vi "rtout_getTriggerConfig.vi"(0 "connection ID":refnum<k5>, 1 "axis":i32, 2 "tempvalue":bool, 5 "error in":errorcluster) -> (12 "polarity":i32, 14 "connection ID":refnum<k5>, 15 "axis_out":i32, 16 "higher":i32, 17 "lower":i32, 18 "epsilon":i32, 19 "error out":errorcluster)   [LabVIEW 2016]
doc: "Get the real time output trigger config"
panel:
  out "params_cluster":cluster{"axis":i32, "tempvalue":bool}
  in  "Params_cluster":cluster{"integer":i32, "boolean":bool}
  in  "results_cluster":T1
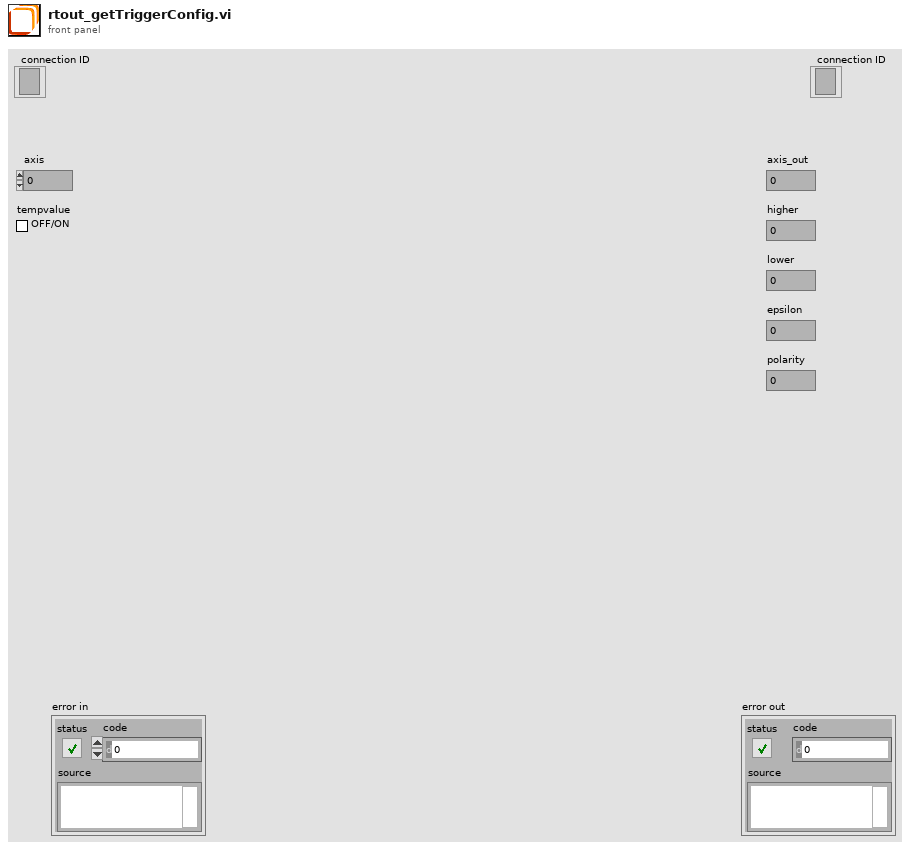
[diagram p1: front panel]
types:
  T1 = cluster{"errNo":i32, "higher":i32, "lower":i32, "epsilon":i32, "polarity":i32}
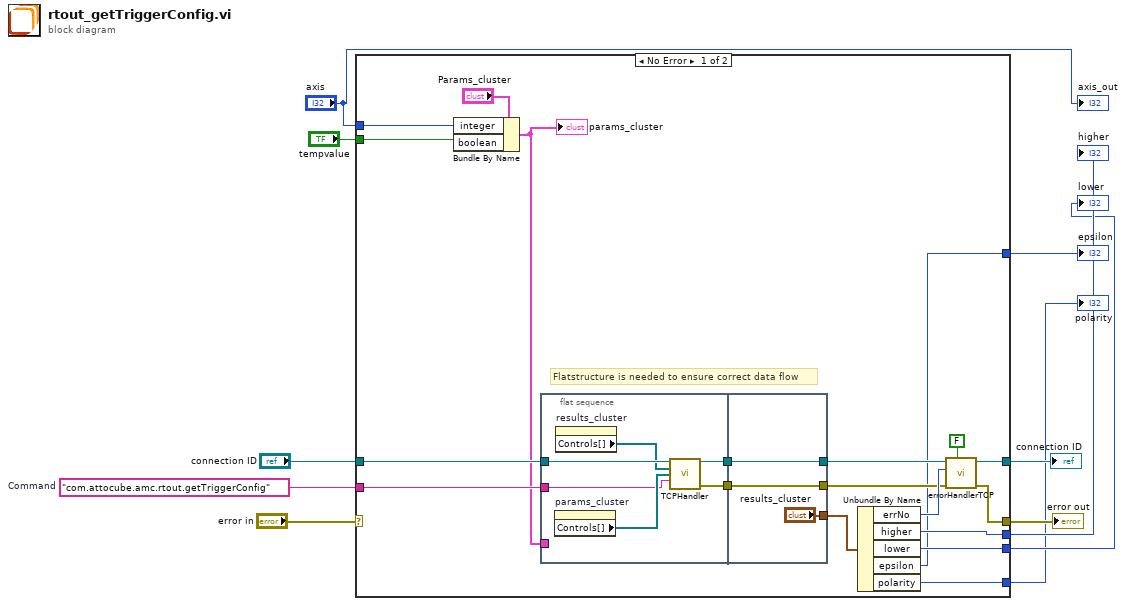
[diagram p0: block diagram]
diagram:
  w7 = "com.attocube.amc.rtout.getTriggerConfig"  # Command
  n1 = case shown="No Error" "error in" {
    selector: "error in" -> [_ w41]
    tunnel: [w28 w41] -> w11
    tunnel: [w30 w40] -> w10
    tunnel: "connection ID" -> [w27 w40]
    tunnel: w7 -> [w21 _]
    tunnel: "axis" -> [w17 _]
    tunnel: "tempvalue" -> [w16 _]
    tunnel: [w15 _] -> w4
    tunnel: [w14 _] -> w3
    tunnel: [w13 _] -> w2
    tunnel: [w12 _] -> w1
    frame No Error {
      # "Flatstructure is needed to ensure correct data flow"
      n2 = Bundle By Name(cluster="Params_cluster", "integer"=w17, "boolean"=w16) -> (w18:cluster{"integer":i32, "boolean":bool})
      "params_cluster" <- w18
      n3 = flat-sequence {
        tunnel: [w35] -> w23
        tunnel: w27 -> [w36]
        tunnel: w21 -> [w32]
        tunnel: [w31] -> w19
        tunnel: w18 -> [_]
        tunnel: ["results_cluster"] -> w24
        tunnel: [w39] -> w26
        tunnel: w23 -> [w39]
        tunnel: [w37] -> w20
        tunnel: w19 -> [w37]
        frame #0 {
          n4 = property on="params_cluster" class="Clust (strict)"() -> ("Controls[]"=w33:refnum<vi>[])  [unwired: 2 in, 2 out]
          n5 = property on="results_cluster" class="Clust (strict)"() -> ("Controls[]"=w34:refnum<vi>[])  [unwired: 2 in, 2 out]
          n6 = call "TCPHandler.vi"("connection ID"=w36, "results_cluster"=w34, "params_cluster"=w33, "method"=w32) -> ("connection ID"=w35:refnum<k5>, "error"=w31:errorcluster)  [unwired: 8 in, 2 out]
        }
        frame #1 {
        }
      }
      n7 = Unbundle By Name(w24) -> ("errNo"=w25:i32, "higher"=w15:i32, "lower"=w14:i32, "epsilon"=w13:i32, "polarity"=w12:i32)
      n8 = call "errorHandlerTCP.vi"("show popup"=FALSE, "error in"=w20, "error number"=w25, "connection ID"=w26) -> ("error out"=w28:errorcluster, "connection ID"=w30:refnum<k5>)  [unwired: 6 in]
    }
    frame Error {
    }
  }
  "error out" <- w11
  "connection ID" <- w10
  "higher" <- w4
  "lower" <- w3
  "epsilon" <- w2
  "polarity" <- w1
  "axis_out" <- "axis"
